vi "Read ProgrammaticInitialization.lvclass.vi"(8 "error in (no error)":errorcluster, 11 "MiddlewareSALThisComponent in":refnum<class "MiddlewareSALThisComponent.lvclass">) -> (0 "error out":errorcluster, 2 "ProgrammaticInitialization.lvclass":refnum<class "ProgrammaticInitialization.lvclass">, 3 "MiddlewareSALThisComponent out":refnum<class "MiddlewareSALThisComponent.lvclass">)   [LabVIEW 2016, in "MiddlewareSALThisComponent.lvclass"]
uses:
  MiddlewareSALThisComponent.lvclass
  ProgrammaticInitialization/ProgrammaticInitialization.lvclass
  MiddlewareSALThisComponent.lvclass/MiddlewareSALThisComponent.ctl
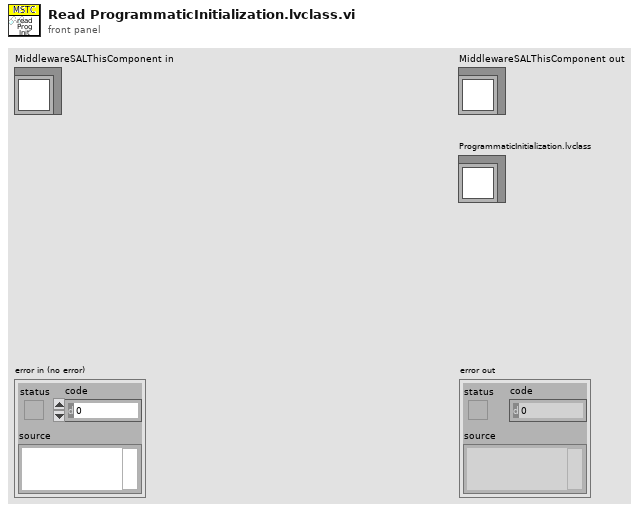
[diagram p1: front panel]
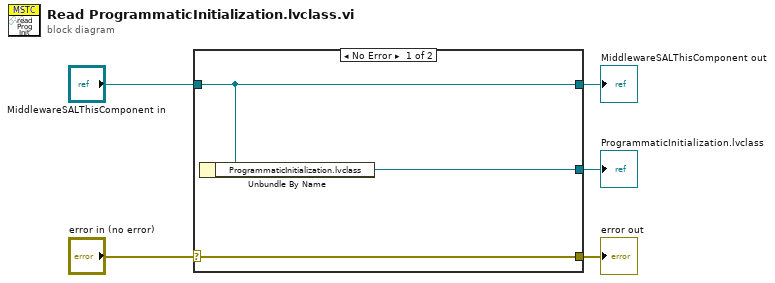
[diagram p0: block diagram]
diagram:
  n1 = case shown="No Error" "error in (no error)" {
    selector: "error in (no error)" -> [w8 w9]
    tunnel: [w8 w9] -> w4
    tunnel: [w7 w10] -> w2
    tunnel: "MiddlewareSALThisComponent in" -> [w7 w10]
    tunnel: [w6 _] -> w1
    frame No Error {
      n2 = Unbundle By Name(w7) -> ("ProgrammaticInitialization.lvclass"=w6:refnum<class "ProgrammaticInitialization.lvclass">)
    }
    frame Error {
    }
  }
  "error out" <- w4
  "MiddlewareSALThisComponent out" <- w2
  "ProgrammaticInitialization.lvclass" <- w1
